vi "Test Initialise.vi"(11 "Test Case In":refnum<class "Renderer Tests.lvclass">) -> (0 "error out":errorcluster, 3 "Test Case Out":refnum<class "Renderer Tests.lvclass">)   [LabVIEW 2021, in "Renderer Tests.lvclass"]
uses:
  Renderer Tests.lvclass
  C:/Program Files (x86)/National Instruments/LabVIEW 2026/vi.lib/Astemes/LUnit/Test Case.lvclass
  <vilib>/Astemes/LUnit/Test Case.lvclass/Test Case.ctl
  Application Specific/Renderer/Renderer.lvclass
  <vilib>/Astemes/LUnit/Test Case.lvclass
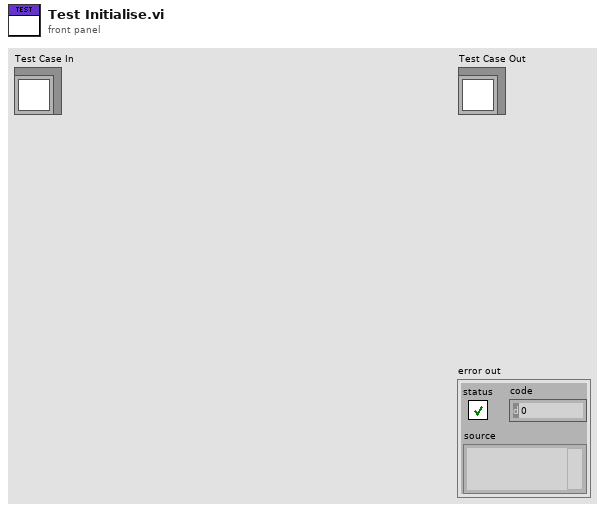
[diagram p1: front panel]
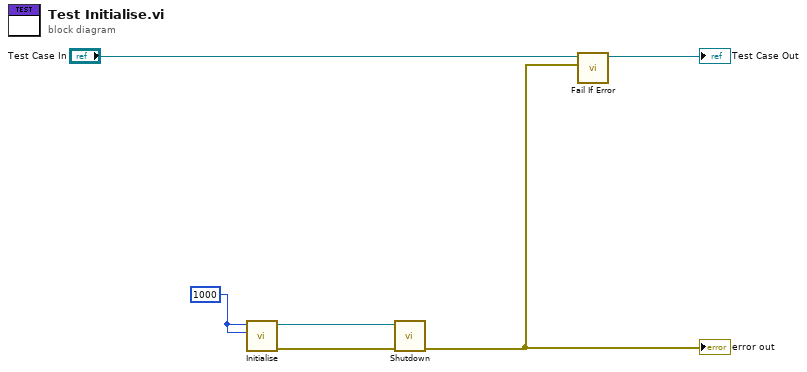
[diagram p0: block diagram]
diagram:
  w1 = 1000 ("Width")
  n1 = call "Initialise.vi"("Height"=w1, "Width"=w1) -> ("error out"=w4:errorcluster, "Renderer out"=w2:refnum<class "Renderer.lvclass">)  [unwired: 8 in]
  n2 = call "Shutdown.vi"("error in (no error)"=w4, "Renderer"=w2) -> ("error out"=w3:errorcluster)  [unwired: 9 in]
  "error out" <- w3
  n3 = call <vilib>:"Fail If Error.vi"("Assert error"=w3, "LUnit Test Case In"="Test Case In") -> ("LUnit Test Case Out"=→"Test Case Out":refnum<class "Renderer Tests.lvclass">)  [unwired: 8 in, 1 out]
